vi "Pack Publish Request.vi"(7 "Publisher ID":string, 9 "Publish Time (Use Current Time)":timestamp, 10 "Data to Publish":variant, 11 "Datum Name":string) -> (3 "PublishRequest":refnum<class "PublishRequest.lvclass">)   [LabVIEW 2017, in "IMediator.lvlib" / "PublishRequest.lvclass"]
uses:
  PublishRequest.lvclass
  PublishRequest.lvclass/PublishRequest.ctl
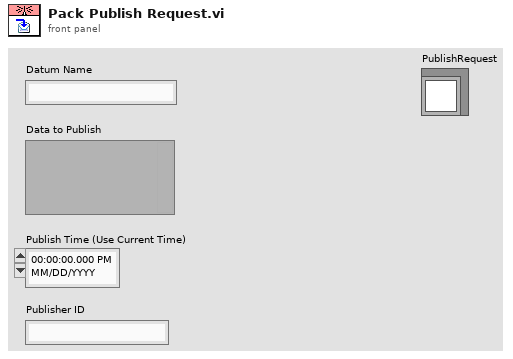
[diagram p1: front panel]
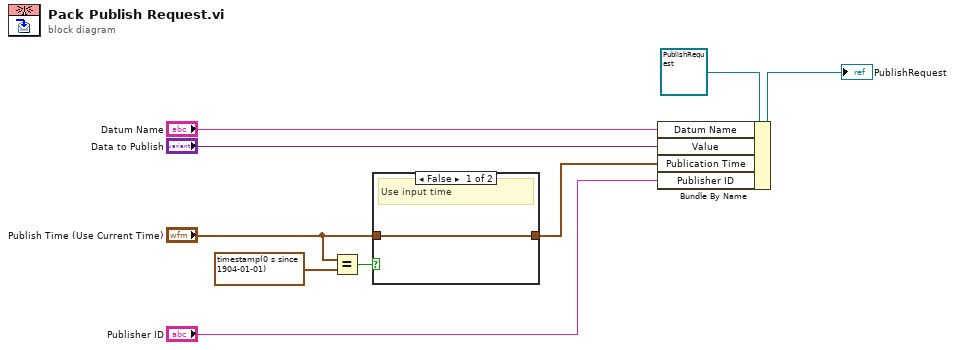
[diagram p0: block diagram]
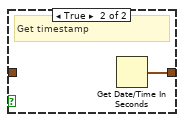
[diagram p2: hidden frame]
diagram:
  n1 = Equal?(x="Publish Time (Use Current Time)", y=timestamp(0 s since 1904-01-01)) -> (x = y?=w4:bool)
  n2 = case shown="False" w4 {
    tunnel: "Publish Time (Use Current Time)" -> [w10 _]
    tunnel: [w10 w11] -> w1
    frame False {
      # "Use input time"
    }
    frame True {
      # "Get timestamp"
      n3 = Get Date/Time In Seconds() -> (seconds since 1Jan1904=w11:timestamp)
    }
  }
  n4 = Bundle By Name(cluster=refnum<class "PublishRequest.lvclass"> refnum ("PublishRequest in"), "Datum Name"="Datum Name", "Value"="Data to Publish", "Publication Time"=w1, "Publisher ID"="Publisher ID") -> (→"PublishRequest":refnum<class "PublishRequest.lvclass">)
